vi "reset_TRIG1.vi"(8 "error in (no error)":errorcluster, 11 "VISA resource name":refnum<visa-resource-name>) -> (0 "error out":errorcluster, 3 "VISA resource name out":refnum<visa-resource-name>)   [LabVIEW 2011]
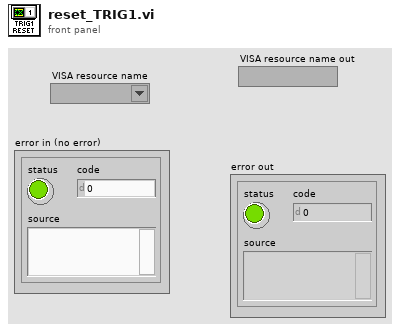
[diagram p1: front panel]
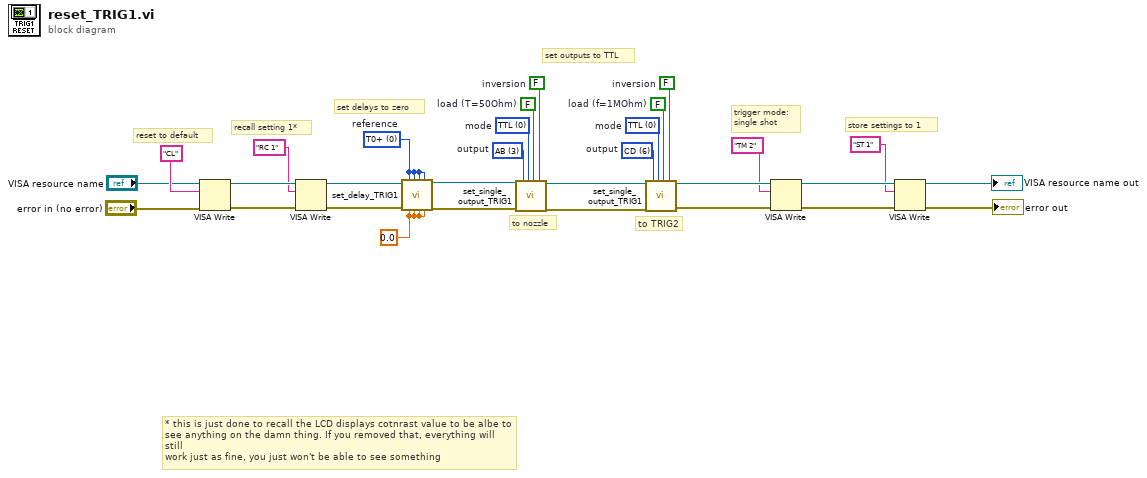
[diagram p0: block diagram]
diagram:
  w13 = FALSE  # inversion
  w14 = FALSE  # load (f=1MOhm)
  w15 = 0 items=["TTL", "NIM", "ECL", "VAR"]  # mode
  w16 = u16 6 items=["T0", "A", "B", "AB", "C", "D", "CD"]  # output
  w17 = FALSE  # inversion
  w18 = FALSE  # load (T=50Ohm)
  w19 = 0 items=["TTL", "NIM", "ECL", "VAR"]  # mode
  w20 = u16 3 items=["T0", "A", "B", "AB", "C", "D", "CD"]  # output
  w23 = 0.0 ("A")
  w24 = u32 0 items=["T0+", "B+", "C+", "D+"]  # reference
  # "store settings to 1"
  # "trigger mode:\nsingle shot"
  # "to TRIG2"
  # "to nozzle"
  # "set outputs to TTL"
  # "* this is just done to recall the LCD displays cotnrast value to be albe to \nsee anything on the damn thing. If you removed that, everything will still\nwork just as fine, you just won't be able to see something"
  # "recall setting 1*"
  # "set delays to zero"
  # "reset to default"
  n1 = VISA Write(VISA resource name="VISA resource name", write buffer="CL", error in (no error)="error in (no error)") -> (VISA resource name out=w29:refnum<visa-resource-name>, error out=w28:errorcluster)  [unwired: 1 out]
  n2 = VISA Write(VISA resource name=w29, write buffer="RC 1", error in (no error)=w28) -> (VISA resource name out=w26:refnum<visa-resource-name>, error out=w25:errorcluster)  [unwired: 1 out]
  n3 = call "set_delay_TRIG1.vi"("VISA resource name"=w26, "error in"=w25, "A ref"=w24, "A"=w23, "B ref"=w24, "B"=w23, "C ref"=w24, "C"=w23, "D ref"=w24, "D"=w23) -> ("VISA resource name out"=w22:refnum<visa-resource-name>, "error out"=w21:errorcluster)  [unwired: 8 in]
  n4 = call "set_single_output_TRIG1.vi"("VISA resource name"=w22, "error in"=w21, "output"=w20, "mode"=w19, "load"=w18, "inversion"=w17) -> ("VISA resource out"=w12:refnum<visa-resource-name>, "error out"=w10:errorcluster)  [unwired: 12 in]
  n5 = call "set_single_output_TRIG1.vi"("VISA resource name"=w12, "error in"=w10, "output"=w16, "mode"=w15, "load"=w14, "inversion"=w13) -> ("VISA resource out"=w8:refnum<visa-resource-name>, "error out"=w11:errorcluster)  [unwired: 12 in]
  n6 = VISA Write(VISA resource name=w8, write buffer="TM 2", error in (no error)=w11) -> (VISA resource name out=w5:refnum<visa-resource-name>, error out=w9:errorcluster)  [unwired: 1 out]
  n7 = VISA Write(VISA resource name=w5, write buffer="ST 1", error in (no error)=w9) -> (VISA resource name out=→"VISA resource name out":refnum<visa-resource-name>, error out=→"error out":errorcluster)  [unwired: 1 out]
